vi "test2_xq1.vi"() -> ()   [LabVIEW 2018]
uses:
  <vilib>/imath/engines/lvmath/Plug In/_Char/NIMS_CH_character datatype.ctl
  <vilib>/imath/engines/lvmath2/RunTimeEngine/RangeToken/NIMS_Range.vi
  <instcachedir>/0/NIMS_Range_846134F467D14A349F7C6CCEF459CDB2.lvgen/NIMS_Range_846134F467D14A349F7C6CCEF459CDB2_000.vi
  <vilib>/imathl/engines/lvmath/Functions/Error Handling/Create Error.vi
  <vilib>/imath/engines/lvmath/Plug In/_Char/NIMS_CH_Character RV to String.vi
  <vilib>/imath/engines/lvmath2/RunTimeEngine/BuiltInFunctions/random/NIMS_random.vi
  <vilib>/imath/engines/lvmath2/RunTimeEngine/IndexRead/NIMS M(S).vi
  <instcachedir>/0/NIMS M(S)_B826C018497E4940AE96BD27B540B6FB.lvgen/NIMS M(S)_B826C018497E4940AE96BD27B540B6FB_000.vi
  <vilib>/imath/engines/lvmath2/RunTimeEngine/ArithmeticOperatorToken/NIMS_ArithmeticOperator_plus.vi
  <instcachedir>/0/NIMS_ArithmeticOperator_plus_DE670E32103C4C10ADF2A97367172B30.lvgen/NIMS_ArithmeticOperator_plus_DE670E32103C4C10ADF2A97367172B30_004.vi
  <vilib>/imath/engines/lvmath2/RunTimeEngine/ErrorHandling/NIMS_Create Error From Enums.vi
  <vilib>/imath/engines/lvmath2/RunTimeEngine/BuiltInFunctions/randnormal/NIMS_randnormal(1,I32).vi
  <vilib>/imath/engines/lvmath2/RunTimeEngine/ErrorHandling/NIMS_Error From Error Code.vi
  <vilib>/imath/engines/lvmath/Functions/Error Handling/MergeErrorsWrapper.vi
  <vilib>/imath/engines/lvmath2/RunTimeEngine/BuiltInFunctions/fft/NIMS_fft(GV).vi
  <instcachedir>/0/NIMS_fft(GV)_4C6467FC22F84E4BA42517A07EF978B0.lvgen/NIMS_fft(GV)_4C6467FC22F84E4BA42517A07EF978B0_000.vi
  <vilib>/imath/engines/lvmath2/RunTimeEngine/BuiltInFunctions/abs/NIMS_abs(signed).vi
  <instcachedir>/0/NIMS_abs(signed)_C4FCB8E6058B49B797C7C8D53CA5F6EC.lvgen/NIMS_abs(signed)_C4FCB8E6058B49B797C7C8D53CA5F6EC_006.vi
  <vilib>/imath/engines/lvmath2/RunTimeEngine/BuiltInFunctions/psd_periodogram/NIMS_psd_periodogram().vi
  <instcachedir>/0/NIMS_psd_periodogram()_02030E41DB254B5B8F4838052F408B46.lvgen/NIMS_psd_periodogram()_02030E41DB254B5B8F4838052F408B46_000.vi
  <vilib>/imath/engines/lvmath2/RunTimeEngine/NodeEndStatement/NIMS_NodeEndStatement_Output.vi
  <instcachedir>/0/NIMS_NodeEndStatement_Output_53EC0D466D134D7ABD903AC30B43404B.lvgen/NIMS_NodeEndStatement_Output_53EC0D466D134D7ABD903AC30B43404B_000.vi
  <instcachedir>/0/NIMS_NodeEndStatement_Output_53EC0D466D134D7ABD903AC30B43404B.lvgen/NIMS_NodeEndStatement_Output_53EC0D466D134D7ABD903AC30B43404B_005.vi
  <vilib>/imath/engines/lvmath2/RunTimeEngine/ErrorHandling/NIMS_Finalize Error.vi
panel:
  out "Sx periodogram":cluster{"BIN":dbl[], "N":dbl[]}(graph)
  out "signal":cluster{"BIN":dbl[], "N":dbl[]}(graph)
  in  "fs":dbl=1000.0
  in  "N":dbl=1024.0
  out "Sx":cluster{"BIN":dbl[], "N":dbl[]}(graph)
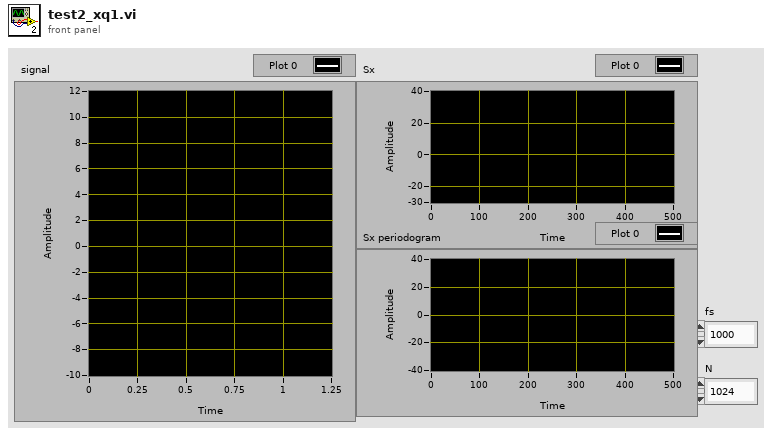
[diagram p1: front panel]
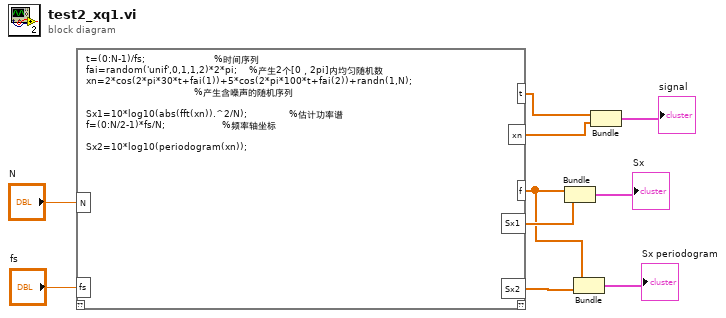
[diagram p0: block diagram]
diagram:
  n1 = mathscript code="t=(0:N-1)/fs;                       %时间序列\nfai=random('unif',0,1,1,2)*2*pi;    %产生2个[0，2pi]内均匀随机数\nxn=2*cos(2*pi*30*t+fai(1))+5*cos(2*pi*100*t+fai(2))+randn(1,N);\n                                    %产生含噪声的随机序列\n\nSx1=10*log10(abs(fft(xn)).^2/N);              %估计功率谱\nf=(0:N/2-1)*fs/N;                   %频率轴坐标\n\nSx2=10*log10(periodogram(xn));"("N"="N", "fs"="fs") -> ("xn"=w4:dbl[], "t"=w5:dbl[], "f"=w1:dbl[], "Sx1"=w7:cdb[], "Sx2"=w2:cdb[])  [unwired: 1 in, 1 out]
  n2 = Bundle("f"=w1, "Sx1"=w7) -> (→"Sx":cluster{"f":dbl[], "Sx1":cdb[]})  [unwired: 1 in]
  n3 = Bundle("f"=w1, "Sx2"=w2) -> (→"Sx periodogram":cluster{"f":dbl[], "Sx2":cdb[]})  [unwired: 1 in]
  n4 = Bundle("t"=w5, "xn"=w4) -> (→"signal":cluster{"t":dbl[], "xn":dbl[]})  [unwired: 1 in]
